vi "Find Clones.vi"(7 "Search Clones Up To":i32=100, 10 "VIs in":string[](array[string]), 11 "Application in":refnum<vi>) -> (2 "VIs (including clones) out":string[](array[string]))   [LabVIEW 2010]
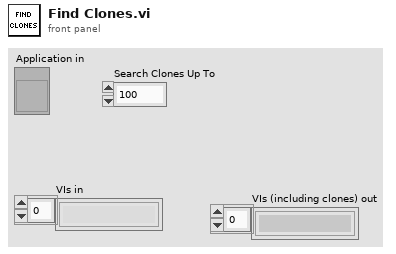
[diagram p1: front panel]
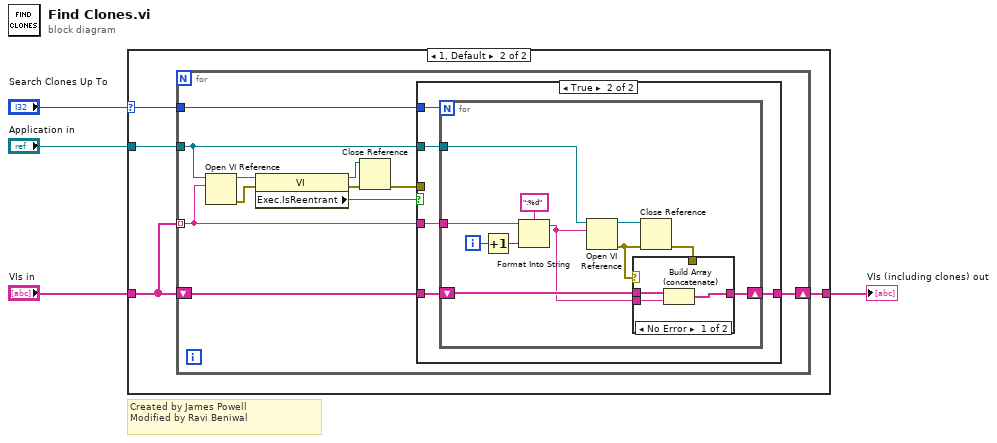
[diagram p0: block diagram]
diagram:
  # "Created by James Powell\nModified by Ravi Beniwal"
  n1 = case shown="1, Default" "Search Clones Up To" {
    selector: "Search Clones Up To" -> [_ w6]
    tunnel: [w5 w9] -> w4
    tunnel: "Application in" -> [_ w8]
    tunnel: "VIs in" -> [w5 w7]
    frame 0 {
    }
    frame 1, Default {
      n2 = for {
        tunnel: w7 -> [w14] mode=indexing
        tunnel: w8 -> [w15]
        shift-right: [w13] -> w9
        shift-left: w7 -> [w11]
        tunnel: w6 -> [w12]
        n3 = Open VI Reference(application reference (local)=w15, vi path=w14) -> (vi reference=w19:refnum<vi>, error out=w20:errorcluster)  [unwired: 4 in]
        n4 = property class="VI"(reference=w19, error in=w20) -> (reference out=w18:refnum<vi>, error out=w17:errorcluster, "Exec.IsReentrant"=w16:bool)
        n5 = Close Reference(reference=w18, error in (no error)=w17) -> (error out=w10:errorcluster)
        n6 = case shown="True" w16 {
          tunnel: w14 -> [_ w26]
          tunnel: w15 -> [_ w25]
          tunnel: w11 -> [w21 w24]
          tunnel: [w21 w23] -> w13
          tunnel: w12 -> [_ w22]
          tunnel: w10 -> [_ _]
          frame False {
          }
          frame True {
            n7 = for {
              N: w22 -> [_]
              tunnel: w26 -> [w37]
              tunnel: w25 -> [w27]
              shift-right: [w32] -> w23
              shift-left: w24 -> [w31]
              i -> [w36]
              n8 = Increment(x=w36) -> (x+1=w28:i32)
              n9 = Format Into String(format string=":%d", initial string=w37, w28) -> (resulting string=w30:string)  [unwired: 1 in, 1 out]
              n10 = Open VI Reference(application reference (local)=w27, vi path=w30) -> (vi reference=w33:refnum<vi>, error out=w34:errorcluster)  [unwired: 4 in]
              n11 = Close Reference(reference=w33, error in (no error)=w34) -> (error out=w29:errorcluster)
              n12 = case shown="No Error" w34 {
                tunnel: [w40 w41] -> w32
                tunnel: w31 -> [w39 w41]
                tunnel: w30 -> [w38 _]
                tunnel: w29 -> [_ _]
                frame No Error {
                  n13 = Build Array (concatenate)(w39, w38) -> (w40:string[])
                }
                frame Error {
                }
              }
            }
          }
        }
      }
    }
  }
  "VIs (including clones) out" <- w4
